vi "Example Graph - Pressure Callback.vi"(4 "Pressure":refnum<user-event>, 5 "Event Data":cluster{"sender":refnum<k24>, "pressure":i32}, 6 "Control Ref":refnum<k24>, 7 "Event Common Data":T1) -> ()   [LabVIEW 2010]
uses:
  C:/tf/play/labview/Tinkerforge.dll
  Tinkerforge.dll
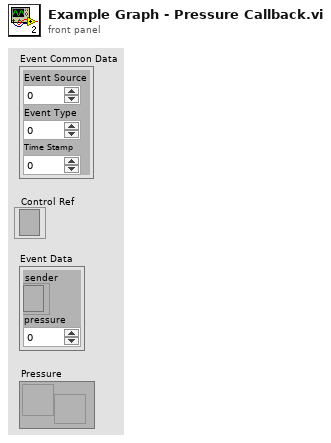
[diagram p1: front panel]
types:
  T1 = cluster{"Event Source":i32, "Event Type":u32, "Time Stamp":u32}
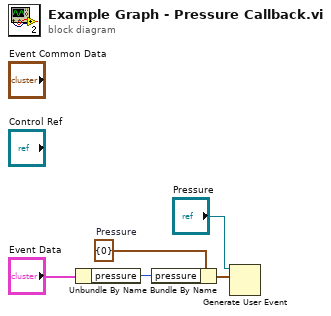
[diagram p0: block diagram]
diagram:
  w4 = cluster{"pressure":i32} {"pressure"=0}  # Pressure
  n1 = Unbundle By Name("Event Data") -> ("pressure"=w3:i32)
  n2 = Bundle By Name(cluster=w4, "pressure"=w3) -> (w2:cluster{"pressure":i32})
  n3 = Generate User Event(user event="Pressure", event data cluster=w2) -> ()  [unwired: 1 in, 2 out]
